vi "Process.vi"(8 "error in (no error)":errorcluster, 10 "Pound in":refnum<class "Pound.lvclass">, 11 "Qbus in":refnum<class "Qbus.lvclass">) -> (0 "error out":errorcluster)   [LabVIEW 2017, in "EmsaDataFlowManager.lvlib"]
uses:
  <vilib>/addons/InsightCM/Devices/Shared/Emsa/EmsaDataFlowManager/EmsaDataFlowManager.lvlib
  <vilib>/addons/Qbus/Qbus.lvclass
  <vilib>/NI/Software Watchdog/Pound/Pound.lvclass
  <vilib>/addons/InsightCM/Devices/Shared/Emsa/EmsaDataFlowManager/controls/config.ctl
  <vilib>/addons/TimerProcess/controls/taskType.ctl
  <vilib>/addons/InsightCM/Devices/Shared/Common/DataFlow/controls/Data.ctl
  <vilib>/addons/InsightCM/Utilities/DataAccessors/controls/wfmSGL_DVR.ctl
  <vilib>/addons/PointValueMap/controls/PointMap.ctl
  <vilib>/addons/InsightCM/Devices/Shared/Common/DataFlow/controls/Type.ctl
  <vilib>/addons/PointValueMap/subVIs/Point_Write_double.vi
  <vilib>/addons/TraceLogger/TraceLogger.lvlib
  <vilib>/NI/Software Watchdog/Watchdog/Watchdog.lvclass
  <vilib>/addons/TimerProcess/TimerProcess.lvlib
  <vilib>/addons/PointValueMap/PointValueMap.lvlib
  <vilib>/addons/InsightCM/Devices/Shared/Common/DataFlow/DataFlow.lvlib
  <vilib>/addons/InsightCM/Utilities/GlobalConfiguration/GlobalConfiguration.lvlib
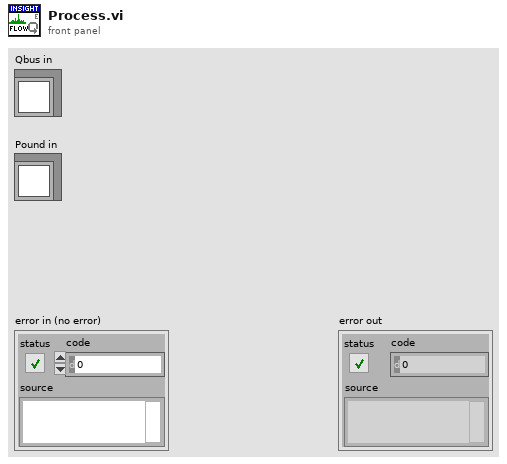
[diagram p1: front panel]
types:
  T1 = typedef "EmsaDataFlowManager.lvlib/config.ctl" = cluster{"poll interval":dbl, "datagroups":string[]}
  T2 = typedef "TimerProcess.lvlib/taskType.ctl" = enum16{"single", "repeat"}
  T3 = typedef "DataFlow.lvlib/Type.ctl" = enum16{"High Rate", "Low Rate", "Burst Mode"}
  T4 = typedef "DataFlow.lvlib/Data.ctl" = cluster{"DataGroup":string, "Waveforms":T5, "Map":T6, "Type":T3}
  T5 = typedef "wfmSGL_DVR.ctl" = refnum<data-value>
  T6 = typedef "PointValueMap.lvlib/PointMap.ctl" = refnum<data-value>
  T7 = typedef "R2_DeviceModel.ctl" = cluster{"Device":T8, "Channels":T16[], "Tags":T18[]}
  T8 = typedef "R2_Device.ctl" = cluster{"Id":string, "Name":string, "DeviceType":string, "HardwareName":string, "IpAddress":string, "HardwareInfo":T9[], "ApplicationType":string, "ApplicationVersion":string, "EquipmentIds":string[], "ConfigurationVersion":string, "State":T10, "Properties":T9[], "DataGroups":T11[], "BurstModeTrigger":T15}
  T9 = typedef "KeyValuePair.ctl" = cluster{"Key":string, "Value":string}
  T10 = typedef "DeviceState.ctl" = cluster{"Disabled":bool}
  T11 = typedef "R2_DataGroup.ctl" = cluster{"Name":string, "OperatingStates":T12[], "Properties":T9[], "EquipmentIds":string[], "AssetNodeId":string}
  T12 = typedef "OperatingState.ctl" = cluster{"Name":string, "Properties":T9[], "Triggers":T13[]}
  T13 = typedef "Trigger.ctl" = cluster{"Type":string, "Expression":string, "Conditions":T14[]}
  T14 = typedef "Condition.ctl" = cluster{"Source":string, "Type":string, "Operator":string, "CompareTo":string, "DwellSeconds":dbl}
  T15 = typedef "BurstModeTrigger.ctl" = cluster{"Trigger":T13, "SampleRate":string, "AcquisitionLength":string}
  T16 = typedef "R2_Channel.ctl" = cluster{"Id":string, "DeviceId":string, "Name":string, "ChannelType":string, "HardwareKey":string, "HardwareChannel":string, "DataGroup":string, "Keywords":string[], "EquipmentIds":string[], "Properties":T9[], "Metrics":T17[], "AssetNodeId":string, "MeasType":string, "AssetName":string}
  T17 = typedef "Metric.ctl" = cluster{"Id":string, "Name":string, "Unit":string, "Properties":T9[], "MetricDefinitionInstanceId":string}
  T18 = typedef "Tag.ctl" = cluster{"Id":string, "Path":string, "Name":string, "Datatype":string, "Props":T9[], "Keywords":string[]}
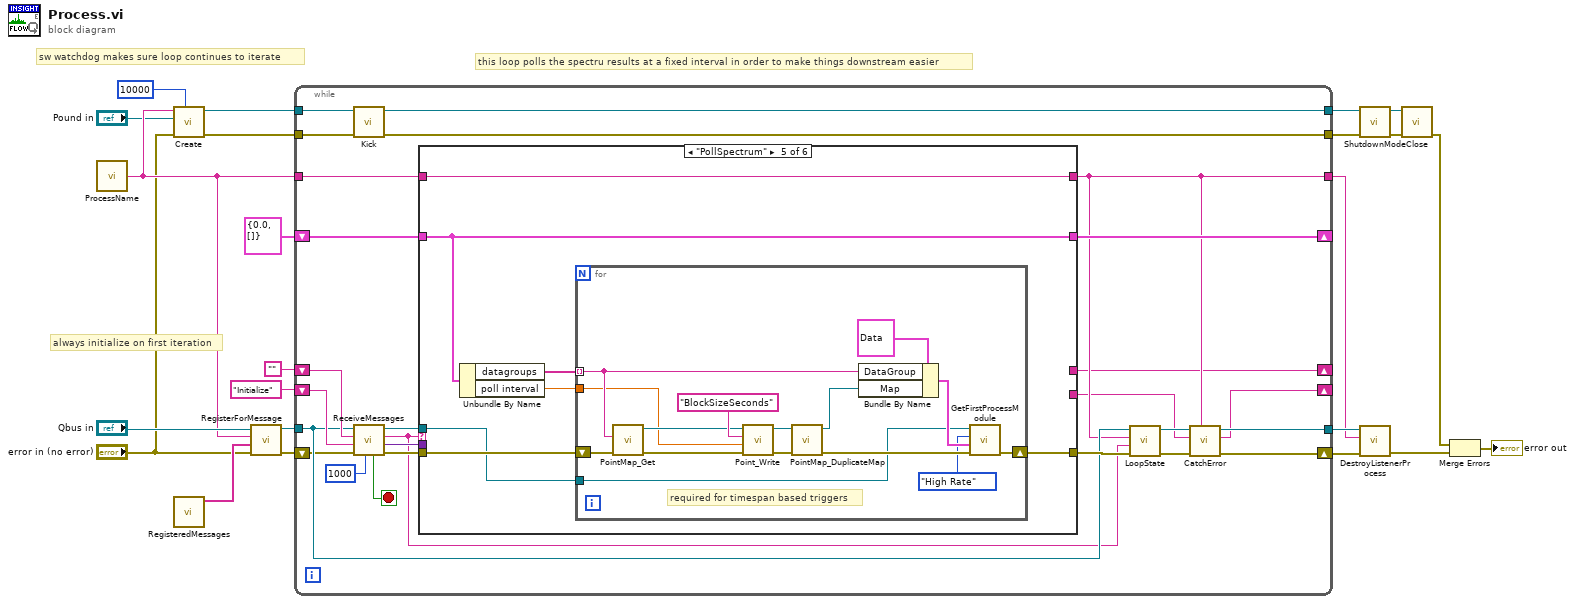
[diagram p0: block diagram]
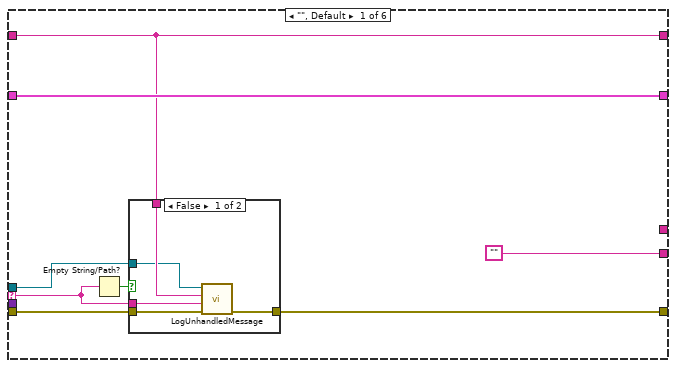
[diagram p2: hidden frame]
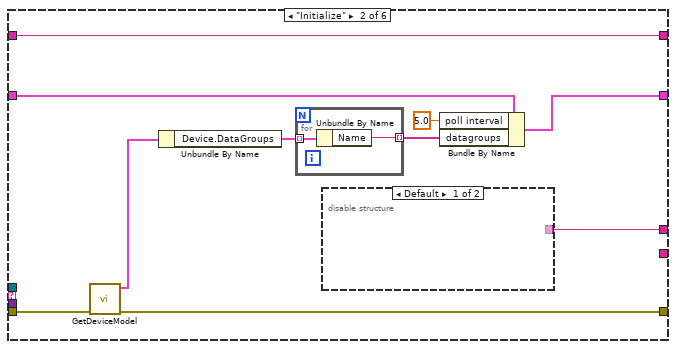
[diagram p4: hidden frame]
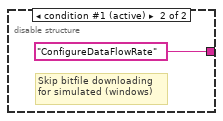
[diagram p5: hidden frame]
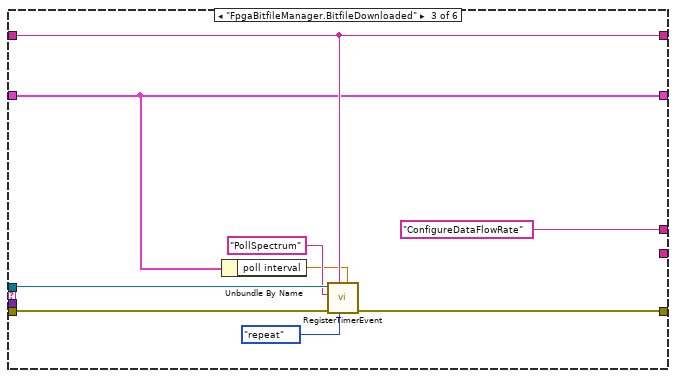
[diagram p6: hidden frame]
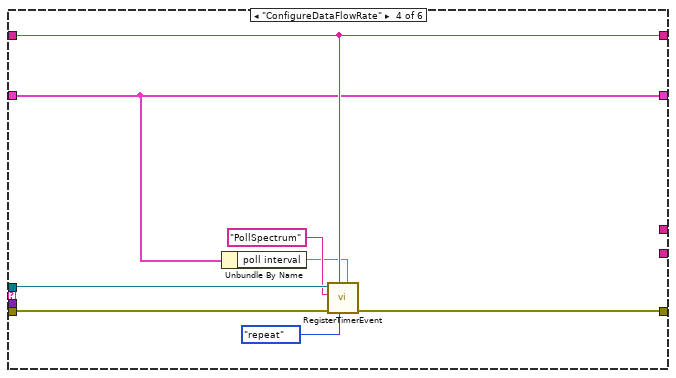
[diagram p7: hidden frame]
diagram:
  # "this loop polls the spectru results at a fixed interval in order to make things downstream easier"
  # "always initialize on first iteration"
  # "sw watchdog makes sure loop continues to iterate"
  n1 = call <vilib>:"ProcessName.vi"() -> ("process name"=w13:string)  [unwired: 5 in]
  n2 = call <vilib>:"Create.vi"("Execution Timeout (ms)"=u32 10000, "error in (no error)"="error in (no error)", "Pound"="Pound in", "Name"=w13) -> ("error out"=w6:errorcluster, "Watchdog"=w12:refnum<data-value>)  [unwired: 6 in]
  n3 = call <vilib>:"RegisteredMessages.vi"() -> ("registered messages"=w14:string[])  [unwired: 11 in]
  n4 = call <vilib>:"RegisterForMessage.vi"("error in (no error)"="error in (no error)", "message names"=w14, "process name"=w13, "Qbus in"="Qbus in") -> ("error in (no error)"=w22:errorcluster, "Qbus out"=w21:refnum<class "Qbus.lvclass">)  [unwired: 6 in]
  n5 = while {
    shift-right: [w24] -> _
    shift-left: "" -> [w48]
    tunnel: w21 -> [w37]
    tunnel: w13 -> [w27]
    tunnel: [w40] -> w19
    tunnel: [w26] -> w18
    shift-right: [w39] -> _
    shift-left: "Initialize" -> [w44]
    shift-right: [w42] -> _
    shift-left: T1 {"poll interval"=0.0, "datagroups"=[]} ("config") -> [w43]
    tunnel: w12 -> [w36]
    tunnel: [w35] -> w8
    tunnel: w6 -> [w34]
    tunnel: [w32] -> w5
    shift-right: [w41] -> w20
    shift-left: w22 -> [w33]
    stop <- w49 stop-if-true
    n6 = call <vilib>:"Kick.vi"("error in (no error)"=w34, "Watchdog"=w36) -> ("error out"=w32:errorcluster, "Watchdog"=w35:refnum<data-value>)  [unwired: 8 in]
    n7 = call <vilib>:"ReceiveMessages.vi"("Timeout(1000)"=1000 ("milliseconds to wait"), "error in (no error)"=w33, "priority action"=w44, "default action"=w48, "Qbus in"=w37) -> ("error out"=w47:errorcluster, "message value"=w45:variant, "action"=w31:string, "Qbus out"=w46:refnum<class "Qbus.lvclass">, "exit"=w49:bool)  [unwired: 2 in]
    n8 = case shown="\"PollSpectrum\"" w31 {
      selector: w31 -> [w54 _ _ _ _ _]
      tunnel: w47 -> [w56 w72 w85 w93 w99 w118]
      tunnel: w46 -> [w52 _ w83 w91 w97 _]
      tunnel: [w55 w71 w84 w92 w98 w118] -> w38
      tunnel: w45 -> [_ _ _ _ _ _]
      tunnel: w43 -> [w57 w68 w78 w86 w96 w117]
      tunnel: [w57 w69 w78 w86 w96 w117] -> w42
      tunnel: [w50 w73 w82 w90 w100 w116] -> w26
      tunnel: w27 -> [w50 w73 w82 w90 w100 w116]
      tunnel: ["" _ _ _ _ _] -> w25
      tunnel: [_ w64 "ConfigureDataFlowRate" ("callback action") _ _ _] -> w24
      frame "", Default {
        n9 = Empty String/Path?(string/path=w54) -> (empty?=w53:bool)
        n10 = case shown="False" w53 {
          tunnel: [w61 w63] -> w55
          tunnel: w56 -> [w62 w63]
          tunnel: w54 -> [w60 _]
          tunnel: w52 -> [w58 _]
          tunnel: w50 -> [w59 _]
          frame False {
            n11 = call <vilib>:"LogUnhandledMessage.vi"("error in (no error)"=w62, "message"=w60, "process"=w59, "Qbus in"=w58) -> ("error out"=w61:errorcluster)  [unwired: 7 in]
          }
          frame True {
          }
        }
      }
      frame "Initialize" {
        n12 = call <vilib>:"GetDeviceModel.vi"("error in (no error)"=w72) -> ("error out"=w71:errorcluster, "device model"=w70:T7)  [unwired: 8 in, 1 out]
        n13 = Unbundle By Name(w70) -> ("Device.DataGroups"=w67:T11[])
        n14 = for {
          tunnel: w67 -> [w76] mode=indexing
          tunnel: [w75] -> w66 mode=indexing
          n15 = Unbundle By Name(w76) -> ("Name"=w75:string)
        }
        n16 = disable-structure shown="Default" {
          disable-tunnel: [_ "ConfigureDataFlowRate" ("callback action")] -> w64
          frame condition #0 {
          }
          frame condition #1 (active) {
            # "Skip bitfile downloading\nfor simulated (windows)"
          }
        }
        n17 = Bundle By Name(cluster=w68, "poll interval"=5.0, "datagroups"=w66) -> (w69:T1)
      }
      frame "FpgaBitfileManager.BitfileDownloaded" {
        n18 = Unbundle By Name(w78) -> ("poll interval"=w79:dbl)
        n19 = call <vilib>:"RegisterTimerEvent.vi"("interval (sec)"=w79, "type"=taskType."repeat", "process name"=w82, "error in (no error)"=w85, "callback action"="PollSpectrum", "qbus in"=w83) -> ("error out"=w84:errorcluster)  [unwired: 4 in, 1 out]
      }
      frame "ConfigureDataFlowRate" {
        n20 = Unbundle By Name(w86) -> ("poll interval"=w87:dbl)
        n21 = call <vilib>:"RegisterTimerEvent.vi"("interval (sec)"=w87, "type"=taskType."repeat", "process name"=w90, "error in (no error)"=w93, "callback action"="PollSpectrum", "qbus in"=w91) -> ("error out"=w92:errorcluster)  [unwired: 4 in, 1 out]
      }
      frame "PollSpectrum" {
        n22 = Unbundle By Name(w96) -> ("datagroups"=w95:string[], "poll interval"=w94:dbl)
        n23 = for {
          shift-right: [w106] -> w98
          shift-left: w99 -> [w115]
          tunnel: w97 -> [w105]
          tunnel: w95 -> [w103] mode=indexing
          tunnel: w94 -> [w102]
          # "required for timespan based triggers"
          n24 = call <vilib>:"PointMap_Get.vi"("error in (no error)"=w115, "Name"=w103) -> ("error out"=w111:errorcluster, "Map Out"=w112:T6)  [unwired: 7 in, 1 out]
          n25 = call-poly <vilib>:"Point_Write.vi"("Error In"=w111, "Value"=w102, "Tag"="BlockSizeSeconds", "Map"=w112) -> ("Error Out"=w110:errorcluster, "Map Out"=w113:T6)  [unwired: 6 in]
          n26 = call <vilib>:"PointMap_DuplicateMap.vi"("error in (no error)"=w110, "map in"=w113) -> ("error out"=w107:errorcluster, "duplicate map"=w104:T6)  [unwired: 8 in]
          n27 = Bundle By Name(cluster=T4 {"DataGroup"="", "Waveforms"=refnum, "Map"=refnum, "Type"=enum."High Rate"} ("data"), "DataGroup"=w103, "Map"=w104) -> (w108:T4)
          n28 = call <vilib>:"GetFirstProcessModule.vi"("error in (no error)"=w107, "data"=w108, "type"=Type."High Rate" ("Type"), "Qbus in"=w105) -> ("error out"=w106:errorcluster)  [unwired: 6 in, 1 out]
        }
      }
      frame "Exit" {
      }
    }
    n29 = call <vilib>:"LoopState.vi"("error in (no error)"=w38, "loop action"=w31, "process name"=w26, "Qbus in"=w37) -> ("error out"=w29:errorcluster, "Qbus out"=w28:refnum<class "Qbus.lvclass">)  [unwired: 6 in]
    n30 = call <vilib>:"CatchError.vi"("source"=w26, "error in (no error)"=w29, "next action in"=w25, "Qbus in"=w28) -> ("error out"=w41:errorcluster, "next action out"=w39:string, "Qbus out"=w40:refnum<class "Qbus.lvclass">)  [unwired: 5 in]
  }
  n31 = call <vilib>:"ShutdownMode.vi"("error in (no error)"=w5, "Watchdog"=w8) -> ("error out"=w7:errorcluster, "Watchdog"=w9:refnum<data-value>)  [unwired: 8 in]
  n32 = call <vilib>:"DestroyListenerProcess.vi"("error in (no error)"=w20, "process name"=w18, "Qbus in"=w19) -> ("error in (no error)"=w4:errorcluster)  [unwired: 7 in, 1 out]
  n33 = call <vilib>:"Close.vi"("error in (no error)"=w7, "Watchdog"=w9) -> ("error out"=w3:errorcluster)  [unwired: 9 in]
  n34 = Merge Errors(w3, w4) -> (→"error out":errorcluster)
